vi "Insight_Streaming_Stop.vi"(8 "error in (no error)":errorcluster, 11 "Streaming VI":refnum<vi>) -> (0 "error out":errorcluster)   [LabVIEW 2011]
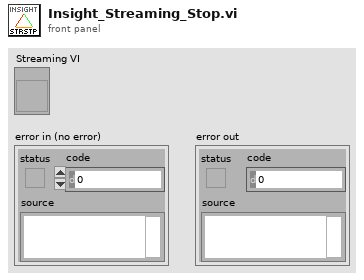
[diagram p1: front panel]
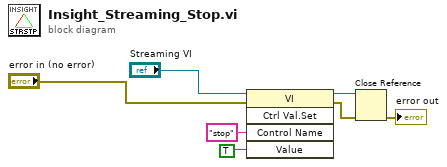
[diagram p0: block diagram]
diagram:
  n1 = invoke class="VI" method="Ctrl Val.Set"(reference="Streaming VI", error in="error in (no error)", "Control Name"="stop", "Value"=TRUE ("stop")) -> (reference out=w5:refnum<vi>, error out=w4:errorcluster)  [unwired: 1 in, 3 out]
  n2 = Close Reference(reference=w5, error in (no error)=w4) -> (error out=→"error out":errorcluster)
